vi "FlatToRichni_xnet_can_bm_api_StopProcessReply.vi"(5 "OutputClusterType":T1, 11 "InputCluster":T3) -> (3 "OutputCluster":T1)   [LabVIEW 2025, in "xnet_can_bus_monitor_api_server.lvlib"]
uses:
  xnet_can_bus_monitor_api_server.lvlib
  ni_xnet_can_bm_api_StopProcessReply_Flat.ctl
  ni_xnet_can_bm_api_ErrorInfo_Flat.ctl
  ni_xnet_can_bm_api_StopProcessReply.ctl
  ni_xnet_can_bm_api_ErrorInfo.ctl
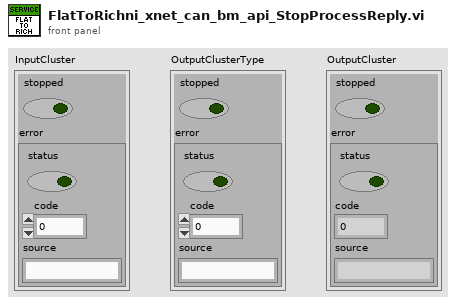
[diagram p1: front panel]
types:
  T1 = typedef "xnet_can_bus_monitor_api_server.lvlib/ni_xnet_can_bm_api_StopProcessReply.ctl" = cluster{"stopped":bool, "error":T2}
  T2 = typedef "xnet_can_bus_monitor_api_server.lvlib/ni_xnet_can_bm_api_ErrorInfo.ctl" = errorcluster
  T3 = typedef "xnet_can_bus_monitor_api_server.lvlib/ni_xnet_can_bm_api_StopProcessReply_Flat.ctl" = cluster{"stopped":bool, "error":T4}
  T4 = typedef "xnet_can_bus_monitor_api_server.lvlib/ni_xnet_can_bm_api_ErrorInfo_Flat.ctl" = errorcluster
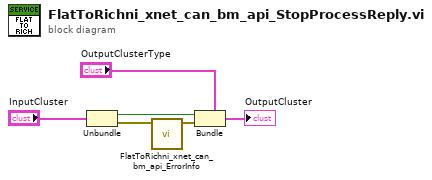
[diagram p0: block diagram]
diagram:
  n1 = Unbundle "Unbundle"("InputCluster") -> ("stopped"=w3:bool, "error"=w2:T4)
  n2 = call "FlatToRichni_xnet_can_bm_api_ErrorInfo.vi"("InputCluster"=w2) -> ("OutputCluster"=w1:T2)  [unwired: 10 in]
  n3 = Bundle "Bundle"(cluster="OutputClusterType", "stopped"=w3, "error"=w1) -> (→"OutputCluster":T1)
